vi "PCO_RecorderStartRecord.vi"(8 "error in (no error)":errorcluster {"code" format="%x"}, 10 "phCam":u64, 11 "phRec":u64) -> (0 "error out":errorcluster {"code" format="%x"}, 2 "ErrorMessage":i32 format="%x", 3 "phRec out":u64)   [LabVIEW 2020, in "Recorder.lvlib"]
doc: "<b>Description:</b>\nThis function starts the recording either for a specific camera or for all cameras (if NULL is transferred as camera handle).\n\n<b>Supported camera type:</b>\nAll cameras"
uses:
  Recorder.lvlib
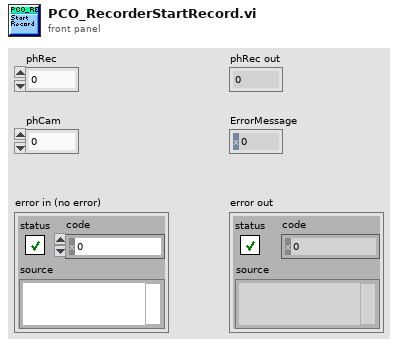
[diagram p1: front panel]
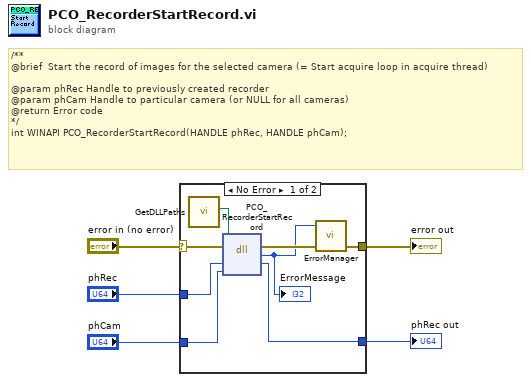
[diagram p0: block diagram]
diagram:
  # "/**\n@brief \tStart the record of images for the selected camera (= Start acquire loop in acquire thread)\n\n@param phRec Handle to previously created recorder\n@param phCam Handle to particular camera (or NULL for all cameras)\n@return Error code\n*/\nint WINAPI PCO_RecorderStartRecord(HANDLE phRec, HANDLE phCam);"
  n1 = case shown="No Error" "error in (no error)" {
    selector: "error in (no error)" -> [w10 w15]
    tunnel: "phRec" -> [w13 w14]
    tunnel: [w12 w14] -> w4
    tunnel: "phCam" -> [w11 _]
    tunnel: [w9 w15] -> w2
    frame No Error {
      n2 = call "GetDLLPaths.vi"() -> ("PCO_Recorder_Path"=w6:path)  [unwired: 9 in, 2 out]
      n3 = dll-call lib="?" fn="PCO_RecorderStartRecord"(path in=w6, error in=w10, "phRec"=w13, "phCam"=w11) -> (error out=w8:errorcluster, "return type"=w7:i32, "phRec"=w12:u64)  [unwired: 2 in, 1 out]
      "ErrorMessage" <- w7
      n4 = call "ErrorManager.vi"("error in (no error)"=w8, "error code"=w7) -> ("error out"=w9:errorcluster)  [unwired: 3 in]
    }
    frame Error {
    }
  }
  "phRec out" <- w4
  "error out" <- w2
